vi "Get FIFO Offsets by Name.vi"(6 "offset":i32, 8 "error in (no error)":errorcluster, 9 "HostToTarget FIFOs":string[](array[string]), 10 "TargetToHost FIFOs":string[](array[string]), 11 "bitfile xml in":string) -> (0 "error out":errorcluster, 1 "HostToTarget FIFO Offsets":T1[](array[typedef]), 2 "TargetToHost FIFO Offsets":T1[](array[typedef]), 4 "offset past EndTag":i32)   [LabVIEW 2010, in "FPGA Bitfile Utility.lvlib"]
uses:
  <userlib>/_FPGA Interface Advanced Tools/FPGA Bitfile Utility/FPGA Bitfile Utility.lvlib
  <userlib>/_FPGA Interface Advanced Tools/FPGA Bitfile Utility/TypeDefs/FIFO Info.ctl
  <vilib>/rvi/DataTransferAndStorage/Container/Common/niFpgaDataTypeControl.ctl
  <userlib>/_FPGA Interface Advanced Tools/FPGA Bitfile Utility/Get FIFOs.vi
  <vilib>/rvi/Utilities/XML/nirviXML_GetValue.vi
  <vilib>/rvi/Utilities/XML/nirviXML_GetValue_String.vi
  resource/RVI/compilationResultUtilities/niLvFpgaGetDmaChannelInfoFromXML.vi
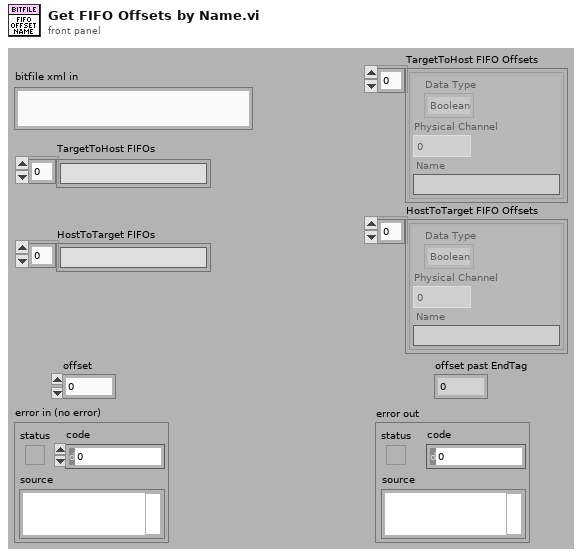
[diagram p1: front panel]
types:
  T1 = typedef "FPGA Bitfile Utility.lvlib/FIFO Info.ctl" = cluster{"Data Type":T2, "Physical Channel":u32, "Name":string}
  T2 = typedef "niFpgaDataTypeControl.ctl" = enum32{"Boolean", "I8", "I16", "I32", "I64", "U8", "U16", "U32", "U64", "FXP", "CustomControl"}
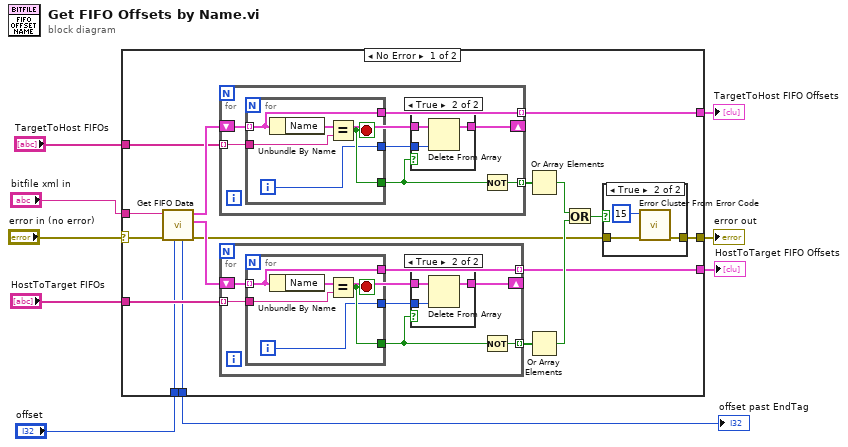
[diagram p0: block diagram]
diagram:
  n1 = case shown="No Error" "error in (no error)" {
    selector: "error in (no error)" -> [w26 w64]
    tunnel: "HostToTarget FIFOs" -> [w21 _]
    tunnel: [w16 _] -> w4
    tunnel: [w15 w64] -> w7
    tunnel: [w14 _] -> w5
    tunnel: "TargetToHost FIFOs" -> [w13 _]
    tunnel: "bitfile xml in" -> [w12 _]
    tunnel: "offset" -> [w11 w63]
    tunnel: [w10 w63] -> w1
    frame No Error {
      n2 = call <userlib>:"Get FIFO Data.vi"("offset"=w11, "error in (no error)"=w26, "bitfile xml in"=w12) -> ("error out"=w17:errorcluster, "HostToTargetFIFOs"=w22:T1[], "TargetToHost FIFOs"=w25:T1[], "offset past EndTag"=w10:i32)  [unwired: 5 in]
      n3 = for {
        tunnel: w13 -> [w53] mode=indexing
        tunnel: [w52] -> w16 mode=indexing
        tunnel: [w51] -> w24 mode=indexing
        shift-right: [w50] -> _
        shift-left: w25 -> [w49]
        n4 = for {
          tunnel: w49 -> [w60] mode=indexing
          tunnel: w53 -> [w61]
          tunnel: [w60] -> w52
          tunnel: [w59] -> w48
          tunnel: [w58] -> w47
          i -> [w58]
          stop <- w59 stop-if-true
          n5 = Unbundle By Name(w60) -> ("Name"=w62:string)
          n6 = Equal?(x=w62, y=w61) -> (x = y?=w59:bool)
        }
        n7 = case shown="True" w48 {
          tunnel: w49 -> [w54 w57]
          tunnel: [w54 w56] -> w50
          tunnel: w47 -> [_ w55]
          frame False {
          }
          frame True {
            n8 = Delete From Array(array=w57, index=w55) -> (array with subset deleted=w56:T1[])  [unwired: 1 in, 1 out]
          }
        }
        n9 = Not(x=w48) -> (.not. x?=w51:bool)
      }
      n10 = for {
        tunnel: w21 -> [w37] mode=indexing
        tunnel: [w36] -> w14 mode=indexing
        tunnel: [w35] -> w23 mode=indexing
        shift-right: [w34] -> _
        shift-left: w22 -> [w33]
        n11 = for {
          tunnel: w33 -> [w44] mode=indexing
          tunnel: w37 -> [w45]
          tunnel: [w44] -> w36
          tunnel: [w43] -> w31
          tunnel: [w42] -> w32
          i -> [w42]
          stop <- w43 stop-if-true
          n12 = Unbundle By Name(w44) -> ("Name"=w46:string)
          n13 = Equal?(x=w46, y=w45) -> (x = y?=w43:bool)
        }
        n14 = case shown="True" w31 {
          tunnel: w33 -> [w38 w41]
          tunnel: [w38 w40] -> w34
          tunnel: w32 -> [_ w39]
          frame False {
          }
          frame True {
            n15 = Delete From Array(array=w41, index=w39) -> (array with subset deleted=w40:T1[])  [unwired: 1 in, 1 out]
          }
        }
        n16 = Not(x=w31) -> (.not. x?=w35:bool)
      }
      n17 = Or Array Elements(Boolean array=w24) -> (logical OR=w20:bool)
      n18 = Or Array Elements(Boolean array=w23) -> (logical OR=w19:bool)
      n19 = Or(x=w20, y=w19) -> (x .or. y?=w18:bool)
      n20 = case shown="True" w18 {
        tunnel: w17 -> [w27 w29]
        tunnel: [w27 w28] -> w15
        frame False {
        }
        frame True {
          n21 = call <vilib>:"Error Cluster From Error Code.vi"("error in (no error)"=w29, "error code (0)"=15) -> ("error out"=w28:errorcluster)  [unwired: 7 in]
        }
      }
    }
    frame Error {
    }
  }
  "error out" <- w7
  "HostToTarget FIFO Offsets" <- w5
  "TargetToHost FIFO Offsets" <- w4
  "offset past EndTag" <- w1
